vi "GetData.vi"(11 "data":dbl[][](array[numeric])) -> (1 "mean 405":dbl, 2 "mean 470":dbl, 3 "F470-F405/F405":dbl)   [LabVIEW 2018]
uses:
  <vilib>/Analysis/baseanly.llb/Mean (DBL).vi
  <vilib>/Analysis/NI_AALBase.lvlib
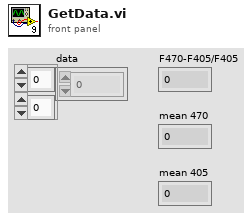
[diagram p1: front panel]
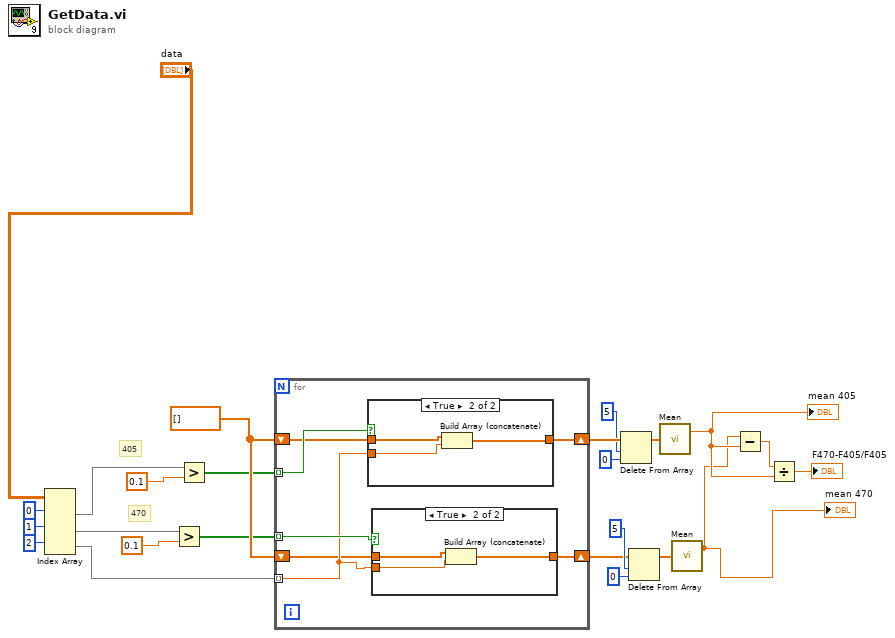
[diagram p0: block diagram]
diagram:
  w22 = dbl[] []
  # "470"
  # "405"
  n1 = Index Array(array="data", index (row) #1=0 ("index (row)"), index (row) #2=1 ("index (row)"), index (row) #3=2 ("index (row)")) -> (element #1=w15:dbl[], element #2=w16:dbl[], element #3=w21:dbl[])  [unwired: 3 in]
  n2 = Greater?(x=w16, y=0.1) -> (0:w20:bool[])
  n3 = Greater?(x=w15, y=0.1) -> (0:w19:bool[])
  n4 = for {
    tunnel: w19 -> [w31] mode=indexing
    tunnel: w20 -> [w30] mode=indexing
    tunnel: w21 -> [w29] mode=indexing
    shift-right: [w28] -> w11
    shift-left: w22 -> [w26]
    shift-right: [w27] -> w5
    shift-left: w22 -> [w25]
    n5 = case shown="True" w31 {
      tunnel: w29 -> [_ w39]
      tunnel: [w36 w38] -> w28
      tunnel: w26 -> [w36 w37]
      frame False {
      }
      frame True {
        n6 = Build Array (concatenate)(w37, w39) -> (w38:dbl[])
      }
    }
    n7 = case shown="True" w30 {
      tunnel: w29 -> [_ w35]
      tunnel: [w32 w34] -> w27
      tunnel: w25 -> [w32 w33]
      frame False {
      }
      frame True {
        n8 = Build Array (concatenate)(w33, w35) -> (w34:dbl[])
      }
    }
  }
  n9 = Delete From Array(array=w11, length=5, index=0) -> (array with subset deleted=w10:dbl[])  [unwired: 1 out]
  n10 = Delete From Array(array=w5, length=5, index=0) -> (array with subset deleted=w4:dbl[])  [unwired: 1 out]
  n11 = call-poly <vilib>:"Mean.vi"("X"=w10) -> ("mean"=w3:dbl)  [unwired: 1 out]
  "mean 405" <- w3
  n12 = call-poly <vilib>:"Mean.vi"("X"=w4) -> ("mean"=w2:dbl)  [unwired: 1 out]
  "mean 470" <- w2
  n13 = Subtract(x=w2, y=w3) -> (x-y=w1:dbl)
  n14 = Divide(x=w1, y=w3) -> (x/y=→"F470-F405/F405":dbl)
